vi "PH_ImageCalibrator.panel.vi"(0 "object ref":refnum<vi>, 5 "error in (no error)":errorcluster) -> (19 "error out":errorcluster)   [LabVIEW 2014, in "PH_ImageCalibrator.lvlib"]
doc: "The voltage measured by a device on high potential is represented by a frequency given out by a Beckhoff Klemme. This VI transforms it back into a voltage which wich is written to a memory tag. This value is indicated. In case of no connection (not mounted or bad tag value) or internal problems \"99999\" apears.\n\n\"Exit\" closes the GUI while \"Delete Instance\" additionally destroys the Instance.\n\n\n\nLicense Agreement for this software:\n\nCopyright (C)\nGesellschaft für Schwerionenforschung, GSI\nPlanckstr. 1\n64291 Darmstadt\nGermany\n\nContact: D.Beck@gsi.de \n\nThis program is free software; you can redistribute it and/or modify it under the terms of the GNU General Public License as published by the Free Software Foundation; either version 2 of the license, or (at your option) any later version.\n\nThis program is distributed in the hope that it will be useful, but WITHOUT ANYW ARRANTY; without even the implied warranty of MERCHANTABILITY or FITNESS FOR A PARTICULAR PURPOSE. See the GNU General License for more details (http://www.gnu.org).\n\nGesellschaft für Schwerionenforschung, GSI\nPlanckstr. 1, 64291 Darmstadt, Germany\nFor all questions and ideas contact: M.Richter@gsi.de, H.Brand@gsi.de or D.Beck@gsi.de.\nLast update: 18-DEC-2002"
uses:
  PH_ImageCalibrator.lvlib
  PH_Img_BaseClass/PH_Img_BaseClass.Palette.ctl
  PH_Img_BaseClass/PH_Img_BaseClass.GUI Refs.ctl
  CSCore/BaseSM/BaseSM.lvlib
  PH_Common/PH_Common.lvlib
  PH_Img_BaseClass/PH_Img_BaseClass.lvlib
  CSCore/CSSystem/CSSystemLib/CSSystemLib.lvlib
  PH_Class/PH_Class.lvlib
panel:
  in  "Timeout Set":i32 caption="ms"
  in  "Palette":T1 items=["Grey", "Binary", "Gradient", "Rainbow", "Temperature"]
  out "Timeout":u32(colorbox)=16860
  out "Image":T2(plugin-control)
  in  "Length [mm]":dbl
  in  "Energy [mJ]":dbl
  out "Dialog":string
  in  "Repeat":bool
  in  "Skip":bool
  in  "Cancel":bool
  in  "OK":bool
  in  "Available Cams":u16(ring)
  in  "Delete":bool
  # "PCS"
  # "3.40"
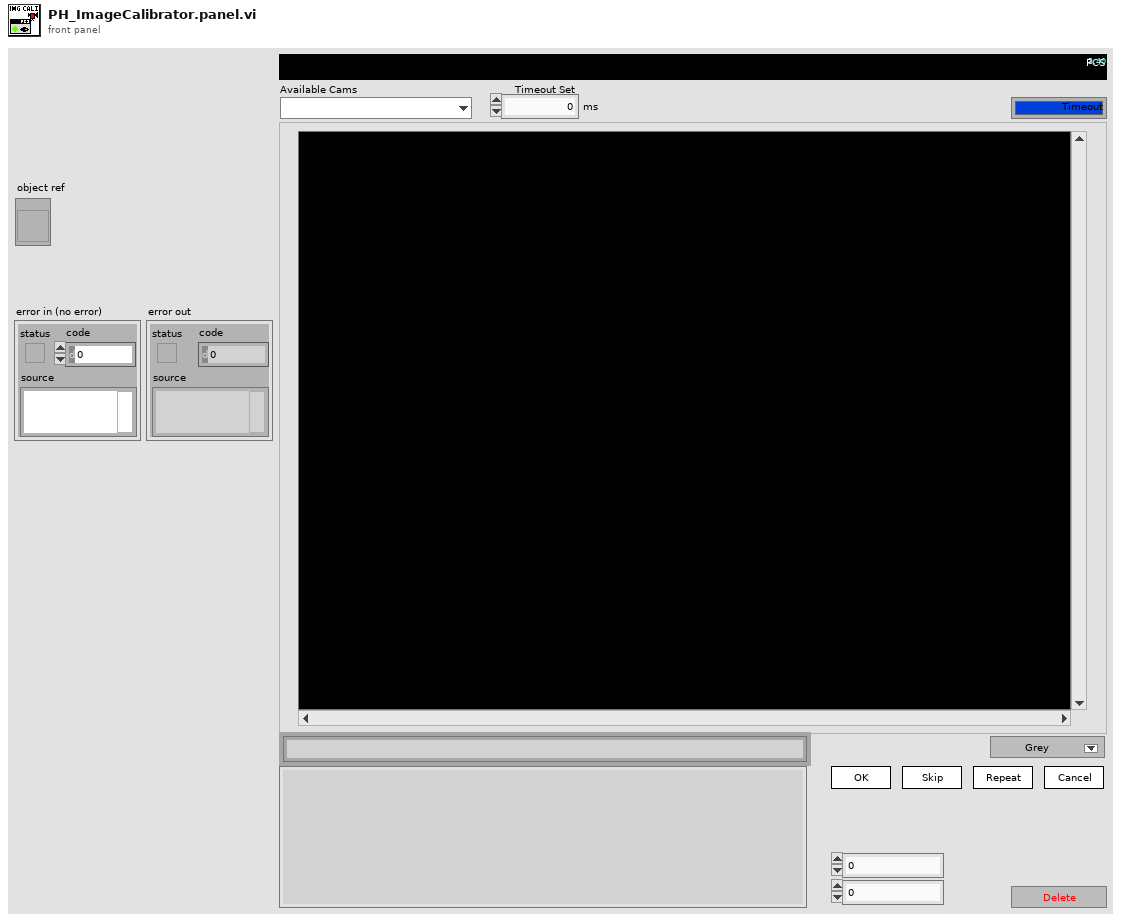
[diagram p1: front panel]
types:
  T1 = typedef "PH_Img_BaseClass.lvlib/PH_Img_BaseClass.Palette.ctl" = i32
  T2 = typedef "IMAQ Image.ctl" = refnum<image>
  T3 = typedef "PH_Img_BaseClass.lvlib/PH_Img_BaseClass.GUI Refs.ctl" = cluster{"Timeout":refnum<vi>, "Image":refnum<vi>, "Palette":refnum<vi>, "Timeout Set":refnum<vi>}
  T4 = typedef "PH_ImageCalibrator.lvlib/PH_ImageCalibrator.i attribute.ctl" = cluster{"GUI Refs":cluster{"Available Cams":refnum<vi>, "OK":refnum<vi>, "Skip":refnum<vi>, "Repeat":refnum<vi>, "Cancel":refnum<vi>, "Length [mm]":refnum<vi>, "Energy [mJ]":refnum<vi>, "Dialog":refnum<vi>}, "Cam instances":string[], "Dark Pics":cluster{"#":i32, "BI taken":bool}, "Lin Cali":cluster{"Distance [Pixel]":dbl, "Distance [mm]":dbl, "Lin Cali Factor [mm/Pixel]":dbl}, "Energy Cali":cluster{"Pixelsum":dbl, "Energy [mJ]":dbl, "Energy Cali factor [mJ/Pixelsum]":dbl, "Underground subtracted?":bool, "#":i32}, "Images":cluster{"Background":T2, "Energy":T2}}
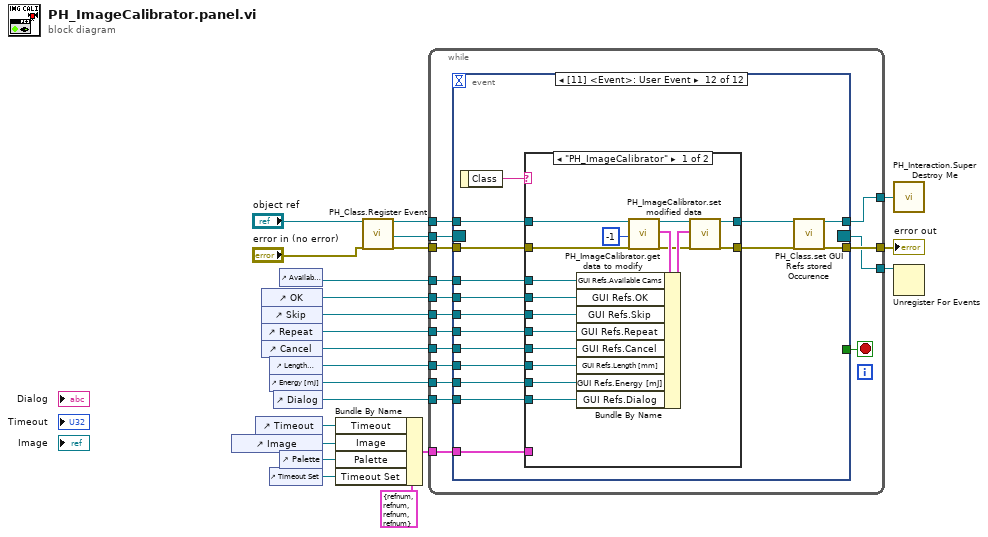
[diagram p0: block diagram]
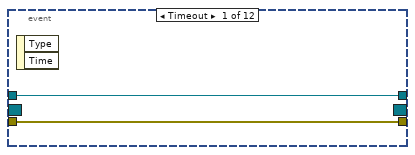
[diagram p2: hidden frame]
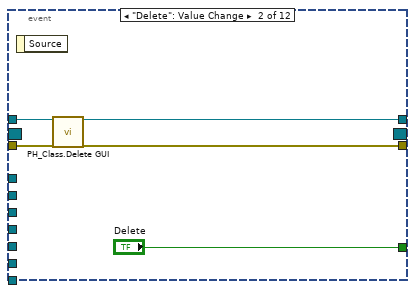
[diagram p3: hidden frame]
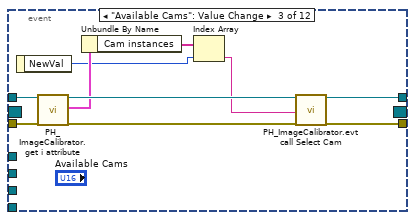
[diagram p4: hidden frame]
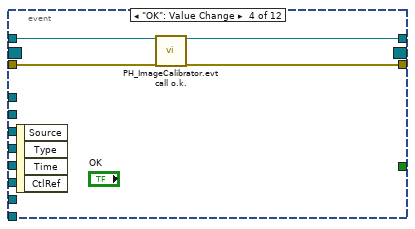
[diagram p5: hidden frame]
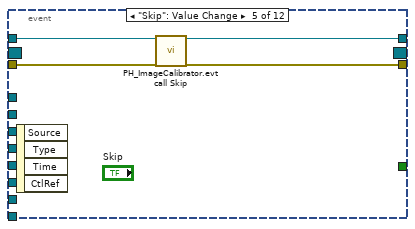
[diagram p6: hidden frame]
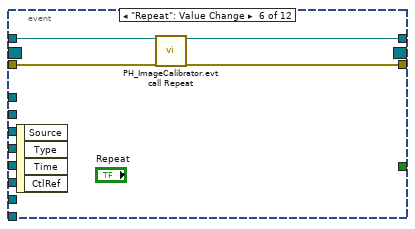
[diagram p7: hidden frame]
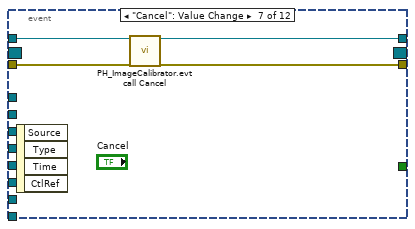
[diagram p8: hidden frame]
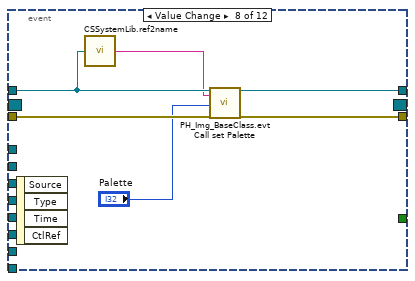
[diagram p9: hidden frame]
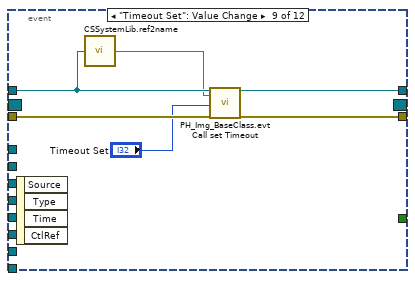
[diagram p10: hidden frame]
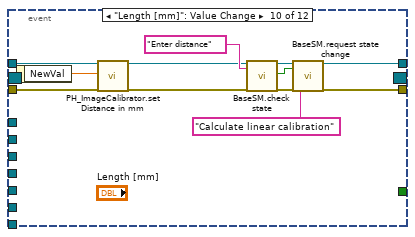
[diagram p11: hidden frame]
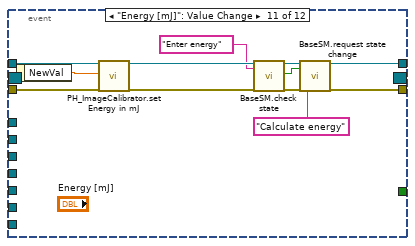
[diagram p12: hidden frame]
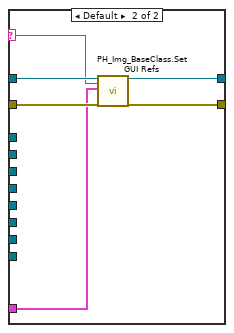
[diagram p13: hidden frame]
diagram:
  n1 = control-ref of="Image"() -> (w19:refnum<vi>)
  n2 = control-ref of="Timeout"() -> (w18:refnum<vi>)
  n3 = control-ref of="OK"() -> (w7:refnum<vi>)
  n4 = control-ref of="Skip"() -> (w6:refnum<vi>)
  n5 = control-ref of="Repeat"() -> (w5:refnum<vi>)
  n6 = control-ref of="Cancel"() -> (w4:refnum<vi>)
  n7 = control-ref of="Length [mm]"() -> (w3:refnum<vi>)
  n8 = control-ref of="Energy [mJ]"() -> (w2:refnum<vi>)
  n9 = control-ref of="Timeout Set"() -> (w16:refnum<vi>)
  n10 = control-ref of="Dialog"() -> (w1:refnum<vi>)
  n11 = control-ref of="Available Cams"() -> (w8:refnum<vi>)
  n12 = control-ref of="Palette"() -> (w17:refnum<vi>)
  n13 = Bundle By Name(cluster=T3 {"Timeout"=refnum, "Image"=refnum, "Palette"=refnum, "Timeout Set"=refnum} ("GUI Refs"), "Timeout"=w18, "Image"=w19, "Palette"=w17, "Timeout Set"=w16) -> (w11:T3)
  n14 = call "PH_Class.Register Event.vi"("i ref in"="object ref", "error in (no error)"="error in (no error)") -> ("i ref out"=w15:refnum<vi>, "Event Registration Refnum"=w13:refnum<event-registration>, "error out"=w14:errorcluster)  [unwired: 15 in]
  n15 = while {
    tunnel: w15 -> [w35]
    tunnel: [w34] -> w22
    tunnel: w14 -> [w37]
    tunnel: [w36] -> w21
    tunnel: w13 -> [w33]
    tunnel: [w32] -> w12
    tunnel: w11 -> [w31]
    tunnel: w8 -> [w30]
    tunnel: w7 -> [w29]
    tunnel: w6 -> [w28]
    tunnel: w5 -> [w27]
    tunnel: w4 -> [w26]
    tunnel: w3 -> [w25]
    tunnel: w2 -> [w24]
    tunnel: w1 -> [w23]
    stop <- w38 stop-if-true
    n16 = event shown="[11] <Event>: User Event" {
      selector: w33 -> [_ _ _ _ _ _ _ _ _ _ _ _]
      dyn-events: [_ _ _ _ _ _ _ _ _ _ _ _] -> w32
      timeout: _ -> [_ _ _ _ _ _ _ _ _ _ _ _]
      tunnel: [_ "Delete" _ _ _ _ _ _ _ _ _ _] -> w38
      tunnel: w35 -> [w39 w44 w52 w59 w63 w67 w70 w74 w80 w95 w107 w123]
      tunnel: w37 -> [w40 w43 w54 w58 w62 w66 w71 w77 w83 w94 w106 w122]
      tunnel: [w40 w41 w55 w57 w61 w65 w69 w76 w82 w84 w99 w108] -> w36
      tunnel: [w39 w42 w46 w56 w60 w64 w68 w75 w81 w86 w101 w109] -> w34
      tunnel: w31 -> [_ _ _ _ _ _ _ _ _ _ _ w121]
      tunnel: w30 -> [_ _ _ _ _ _ _ _ _ _ _ w119]
      tunnel: w29 -> [_ _ _ _ _ _ _ _ _ _ _ w118]
      tunnel: w28 -> [_ _ _ _ _ _ _ _ _ _ _ w117]
      tunnel: w27 -> [_ _ _ _ _ _ _ _ _ _ _ w116]
      tunnel: w26 -> [_ _ _ _ _ _ _ _ _ _ _ w115]
      tunnel: w25 -> [_ _ _ _ _ _ _ _ _ _ _ w114]
      tunnel: w24 -> [_ _ _ _ _ _ _ _ _ _ _ w113]
      tunnel: w23 -> [_ _ _ _ _ _ _ _ _ _ _ w112]
      event Timeout {
        n17 = event-data() -> ()  [unwired: 1 in, 2 out]
      }
      event "Delete": Value Change {
        n18 = event-data() -> ()  [unwired: 1 in, 1 out]
        n19 = call "PH_Class.Delete GUI.vi"("VI in"=w44, "error in (no error)"=w43) -> ("VI out"=w42:refnum<vi>, "error out"=w41:errorcluster)  [unwired: 16 in]
      }
      event "Available Cams": Value Change {
        n20 = event-data() -> ("NewVal"=w48:u16)  [unwired: 1 in]
        n21 = call "PH_ImageCalibrator.get i attribute.vi"("i ref in"=w52, "error in (no error)"=w54) -> ("i ref out"=w51:refnum<vi>, "i attribute"=w50:T4, "error out"=w53:errorcluster)  [unwired: 15 in]
        n22 = Unbundle By Name(w50) -> ("Cam instances"=w49:string[])
        n23 = Index Array(array=w49, index=w48) -> (element=w47:string)
        n24 = call "PH_ImageCalibrator.evt call Select Cam.vi"("i ref in"=w51, "Cam"=w47, "error in"=w53) -> ("i ref out"=w46:refnum<vi>, "error out"=w55:errorcluster)  [unwired: 15 in]
      }
      event "OK": Value Change {
        n25 = event-data() -> ()  [unwired: 1 in, 4 out]
        n26 = call "PH_ImageCalibrator.evt call o.k..vi"("i ref in"=w59, "error in"=w58) -> ("i ref out"=w56:refnum<vi>, "error out"=w57:errorcluster)  [unwired: 16 in]
      }
      event "Skip": Value Change {
        n27 = event-data() -> ()  [unwired: 1 in, 4 out]
        n28 = call "PH_ImageCalibrator.evt call Skip.vi"("i ref in"=w63, "error in"=w62) -> ("i ref out"=w60:refnum<vi>, "error out"=w61:errorcluster)  [unwired: 16 in]
      }
      event "Repeat": Value Change {
        n29 = event-data() -> ()  [unwired: 1 in, 4 out]
        n30 = call "PH_ImageCalibrator.evt call Repeat.vi"("i ref in"=w67, "error in"=w66) -> ("i ref out"=w64:refnum<vi>, "error out"=w65:errorcluster)  [unwired: 16 in]
      }
      event "Cancel": Value Change {
        n31 = event-data() -> ()  [unwired: 1 in, 4 out]
        n32 = call "PH_ImageCalibrator.evt call Cancel.vi"("i ref in"=w70, "error in"=w71) -> ("i ref out"=w68:refnum<vi>, "error out"=w69:errorcluster)  [unwired: 16 in]
      }
      event Value Change {
        n33 = event-data() -> ()  [unwired: 1 in, 4 out]
        n34 = call "CSSystemLib.ref2name.vi"("obj refnum"=w74) -> ("name"=w73:string)
        n35 = call "PH_Img_BaseClass.evt Call set Palette.vi"("i ref in"=w74, "Instance"=w73, "Palette"="Palette", "error in (no error)"=w77) -> ("i ref out"=w75:refnum<vi>, "error out"=w76:errorcluster)  [unwired: 14 in]
      }
      event "Timeout Set": Value Change {
        n36 = event-data() -> ()  [unwired: 1 in, 4 out]
        n37 = call "CSSystemLib.ref2name.vi"("obj refnum"=w80) -> ("name"=w79:string)
        n38 = call "PH_Img_BaseClass.evt Call set Timeout.vi"("i ref in"=w80, "Instance"=w79, "Timeout [ms]"="Timeout Set", "error in (no error)"=w83) -> ("i ref out"=w81:refnum<vi>, "error out"=w82:errorcluster)  [unwired: 14 in]
      }
      event "Length [mm]": Value Change {
        n39 = event-data() -> ("NewVal"=w93:dbl)  [unwired: 1 in]
        n40 = call "PH_ImageCalibrator.set Distance in mm.vi"("i ref in"=w95, "Distance [mm]"=w93, "error in (no error)"=w94) -> ("i ref out"=w87:refnum<vi>, "error out"=w85:errorcluster)  [unwired: 15 in]
        n41 = call "BaseSM.check state.vi"("i ref in"=w87, "requestedState"="Enter distance" ("requested state"), "error in (no error)"=w85) -> ("i ref out"=w92:refnum<vi>, "OK"=w89:bool, "error out"=w91:errorcluster)  [unwired: 11 in, 3 out]
        n42 = call "BaseSM.request state change.vi"("i ref in"=w92, "change"=w89, "error in (no error)"=w91, "requested state"="Calculate linear calibration") -> ("i ref out"=w86:refnum<vi>, "error out"=w84:errorcluster)  [unwired: 12 in, 2 out]
      }
      event "Energy [mJ]": Value Change {
        n43 = event-data() -> ("NewVal"=w105:dbl)  [unwired: 1 in]
        n44 = call "PH_ImageCalibrator.set Energy in mJ.vi"("i ref in"=w107, "Energy [mJ]"=w105, "error in (no error)"=w106) -> ("i ref out"=w104:refnum<vi>, "error out"=w103:errorcluster)  [unwired: 15 in]
        n45 = call "BaseSM.check state.vi"("i ref in"=w104, "requestedState"="Enter energy" ("requested state"), "error in (no error)"=w103) -> ("i ref out"=w102:refnum<vi>, "OK"=w97:bool, "error out"=w100:errorcluster)  [unwired: 11 in, 3 out]
        n46 = call "BaseSM.request state change.vi"("i ref in"=w102, "change"=w97, "error in (no error)"=w100, "requested state"="Calculate energy") -> ("i ref out"=w101:refnum<vi>, "error out"=w99:errorcluster)  [unwired: 12 in, 2 out]
      }
      event User Event {
        n47 = event-data() -> ("Class"=w120:string)  [unwired: 1 in]
        n48 = case shown="\"PH_ImageCalibrator\"" w120 {
          selector: w120 -> [_ w141]
          tunnel: w123 -> [w135 w146]
          tunnel: w122 -> [w134 w145]
          tunnel: [w133 w144] -> w111
          tunnel: [w132 w143] -> w110
          tunnel: w121 -> [_ w142]
          tunnel: w119 -> [w131 _]
          tunnel: w118 -> [w130 _]
          tunnel: w117 -> [w129 _]
          tunnel: w116 -> [w128 _]
          tunnel: w115 -> [w127 _]
          tunnel: w114 -> [w126 _]
          tunnel: w113 -> [w125 _]
          tunnel: w112 -> [w124 _]
          frame "PH_ImageCalibrator" {
            n49 = call "PH_ImageCalibrator.get data to modify.vi"("i ref in"=w135, "ms timeout (10000)"=-1, "error in (no error)"=w134) -> ("i ref out"=w136:refnum<vi>, "i attribute"=w139:T4, "error out"=w137:errorcluster)  [unwired: 13 in, 1 out]
            n50 = Bundle By Name(cluster=w139, "GUI Refs.Available Cams"=w131, "GUI Refs.OK"=w130, "GUI Refs.Skip"=w129, "GUI Refs.Repeat"=w128, "GUI Refs.Cancel"=w127, "GUI Refs.Length [mm]"=w126, "GUI Refs.Energy [mJ]"=w125, "GUI Refs.Dialog"=w124) -> (w140:T4)
            n51 = call "PH_ImageCalibrator.set modified data.vi"("i ref in"=w136, "i attribute"=w140, "error in (no error)"=w137) -> ("i ref out"=w133:refnum<vi>, "error out"=w132:errorcluster)  [unwired: 15 in]
          }
          frame Default {
            n52 = call "PH_Img_BaseClass.Set GUI Refs.vi"("i ref in"=w146, "Class"=w141, "GUI Refs"=w142, "error in (no error)"=w145) -> ("i ref out"=w144:refnum<vi>, "error out"=w143:errorcluster)  [unwired: 14 in]
          }
        }
        n53 = call "PH_Class.set GUI Refs stored Occurence.vi"("i ref in"=w111, "error in (no error)"=w110) -> ("i ref out"=w109:refnum<vi>, "error out"=w108:errorcluster)  [unwired: 16 in]
      }
    }
  }
  "error out" <- w21
  n54 = call "PH_Interaction.Super Destroy Me.vi"("i ref out"=w22) -> ()
  n55 = Unregister For Events(event registration refnum=w12) -> ()  [unwired: 1 in, 1 out]
